vi "Manual.vi"(6 "Cluster":T9={"VISA resource name"="", "baud rate "=9600}, 7 "vi reference":refnum<vi>, 8 "error in (no error)":errorcluster, 9 "IOList_280":T1, 10 "TabCtl Refnum":refnum<vi>, 11 "Manual":T4(tab)) -> (0 "error out":errorcluster, 3 "Out reference":refnum<vi>)   [LabVIEW 2015]
uses:
  Control Button/Exit.ctl
  Control Button/Scanner config.ctl
  Galobal variable_TI.vi
  <vilib>/Instr/_visa.llb/VISA Configure Serial Port (Instr).vi
panel:
  out "Array":string[](array[string])
  out "Byte Lenth":i32
  out "error out 2":errorcluster
  out "Manual DO":bool[](array[boolean])
  in  "Stop":T2
  out "NewVal":T3
  in  "Digital Output":T5
  out "Digital Input":T6
  in  "Home Calling M1":bool
  in  "Stop M1":bool
  in  "Direction M1":bool
  in  "SERVO ON CMD M1":bool
  in  "Speed (mm/s) M1":dbl=10.0
  in  "Travel (mm)M1":dbl=5.0
  out "STM1 Done Bit":bool
  in  "Mode M1":i32(ring)=10178 items=["Finite Samples"=10178, "Continuous Samples"=10123, "Hardware Timed Single Point"=12522]
  out "Waveform Chart":dbl(graph)
  out "Analog Input":T7
  out "Error Status":bool
  in  "Scanner config":T8
  out "Read data":string
  out "Boolean":bool
  # "Fixture Slide servo"
  # "Instruction for Servo motor Operate\n(1)  Switch  ON -OFF  of Fixture Slide servo Brake ON Cmd (P0.19)  \n      from Digital Output tab.\n(2) Switch  ON -OFF  of Fixture Slide Servo Direction Command (P0.20)\n      from Digital Output tab."
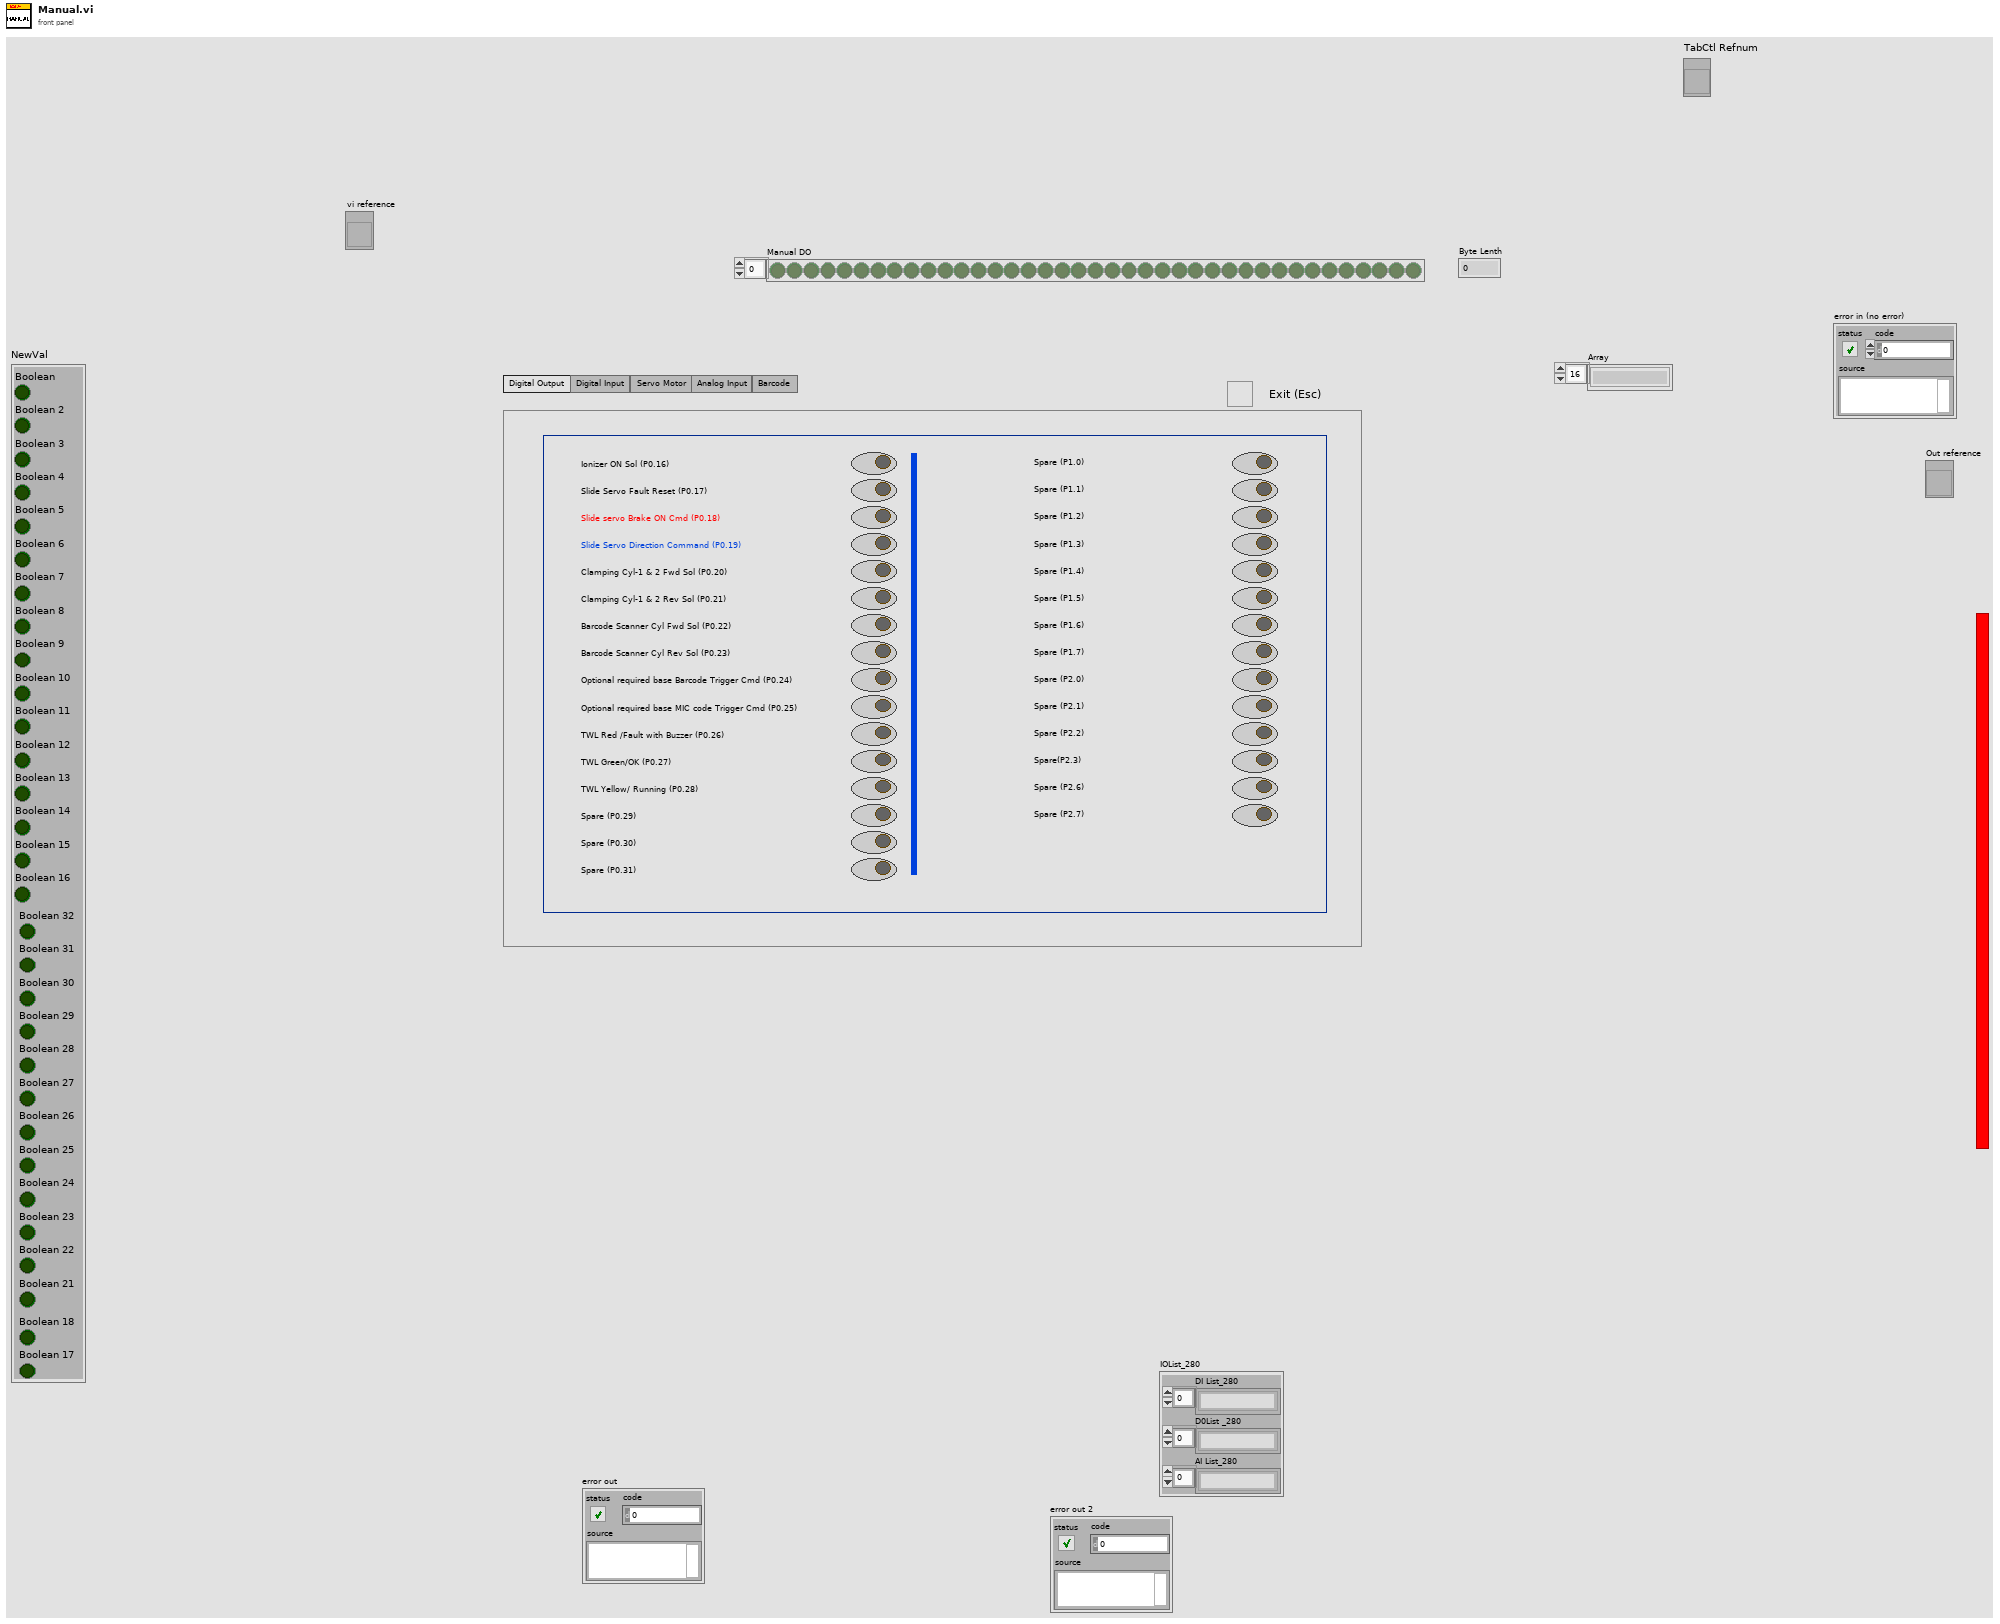
[diagram p1: front panel]
types:
  T1 = cluster{"DI List_280":string[], "D0List _280":string[], "AI List_280":string[]}
  T2 = typedef "Exit.ctl" = bool
  T3 = cluster{"Boolean":bool, "Boolean 2":bool, "Boolean 3":bool, "Boolean 4":bool, "Boolean 5":bool, "Boolean 6":bool, "Boolean 7":bool, "Boolean 8":bool, "Boolean 9":bool, "Boolean 10":bool, "Boolean 11":bool, "Boolean 12":bool, "Boolean 13":bool, "Boolean 14":bool, "Boolean 15":bool, "Boolean 16":bool, "Boolean 17":bool, "Boolean 18":bool, "Boolean 21":bool, "Boolean 22":bool, "Boolean 23":bool, "Boolean 24":bool, "Boolean 25":bool, "Boolean 26":bool, "Boolean 27":bool, "Boolean 28":bool, "Boolean 29":bool, "Boolean 30":bool, "Boolean 31":bool, "Boolean 32":bool}
  T4 = enum32{"Digital Output", "Digital Input", "Servo Motor ", "Analog Input", "Barcode "}
  T5 = cluster{"DO.00":bool, "DO.01":bool, "DO.02":bool, "DO.03":bool, "DO.04":bool, "DO.05":bool, "DO.06":bool, "DO.06":bool, "DO.07":bool, "DO.08":bool, "DO.09":bool, "DO.10":bool, "DO.11":bool, "DO.12":bool, "DO.13":bool, "DO.14":bool, "DO.07 2":bool, "DO.08 2":bool, "DO.09 2":bool, "DO.10 2":bool, "DO.11 2":bool, "DO.12 2":bool, "DO.13 2":bool, "DO.14 2":bool, "DO.00 2":bool, "DO.01 2":bool, "DO.02 2":bool, "DO.03 2":bool, "DO.06 2":bool, "DO.06 3":bool}
  T6 = cluster{"Digital Input":bool, "Digital Input 2":bool, "Digital Input 3":bool, "Digital Input 4":bool, "Digital Input 5":bool, "Digital Input 6":bool, "Digital Input 7":bool, "Digital Input 8":bool, "Digital Input 9":bool, "Digital Input 10":bool, "Digital Input 11":bool, "Digital Input 12":bool, "Digital Input 13":bool, "Digital Input 14":bool, "Digital Input 15":bool, "Digital Input 16":bool, "Digital Input 17":bool, "Digital Input 18":bool, "Digital Input 19":bool, "Digital Input 20":bool, "Digital Input 21":bool, "Digital Input 22":bool, "Digital Input 23":bool, "Digital Input 24":bool, "Digital Input 25":bool, "Digital Input 26":bool, "Digital Input 27":bool, "Digital Input 28":bool, "Digital Input 29":bool, "Digital Input 30":bool, "Digital Input 31":bool, "Digital Input 32":bool, "Digital Input 33":bool, "Digital Input 34":bool, "Digital Input 35":bool, "Digital Input 36":bool, "Digital Input 37":bool, "Digital Input 38":bool, "Digital Input 39":bool}
  T7 = cluster{"Analog Data":dbl, "Analog Data 2":dbl, "Analog Data 3":dbl, "Analog Data 4":dbl, "Analog Data 5":dbl, "Analog Data 6":dbl}
  T8 = typedef "Scanner config.ctl" = bool
  T9 = cluster{"VISA resource name":refnum<visa-resource-name>, "baud rate ":u32}
  T10 = cluster{"Analoge Input[0]":dbl, "Analoge Input[1]":dbl, "Analoge Input[2]":dbl, "Analoge Input[3]":dbl, "Analoge Input[4]":dbl, "Analoge Input[5]":dbl}
  T11 = cluster{"Digital input[0]":bool, "Digital input[1]":bool, "Digital input[2]":bool, "Digital input[3]":bool, "Digital input[4]":bool, "Digital input[5]":bool, "Digital input[6]":bool, "Digital input[7]":bool, "Digital input[8]":bool, "Digital input[9]":bool, "Digital input[10]":bool, "Digital input[11]":bool, "Digital input[12]":bool, "Digital input[13]":bool, "Digital input[14]":bool, "Digital input[15]":bool, "Digital input[16]":bool, "Digital input[17]":bool, "Digital input[18]":bool, "Digital input[19]":bool, "Digital input[20]":bool, "Digital input[21]":bool, "Digital input[22]":bool, "Digital input[23]":bool, "Digital input[24]":bool, "Digital input[25]":bool, "Digital input[26]":bool, "Digital input[27]":bool, "Digital input[28]":bool, "Digital input[29]":bool, "Digital input[30]":bool, "Digital input[31]":bool, "Digital input[32]":bool, "Digital input[33]":bool, "Digital input[34]":bool, "Digital input[35]":bool, "Digital input[36]":bool, "Digital input[37]":bool, "Digital input[38]":bool}
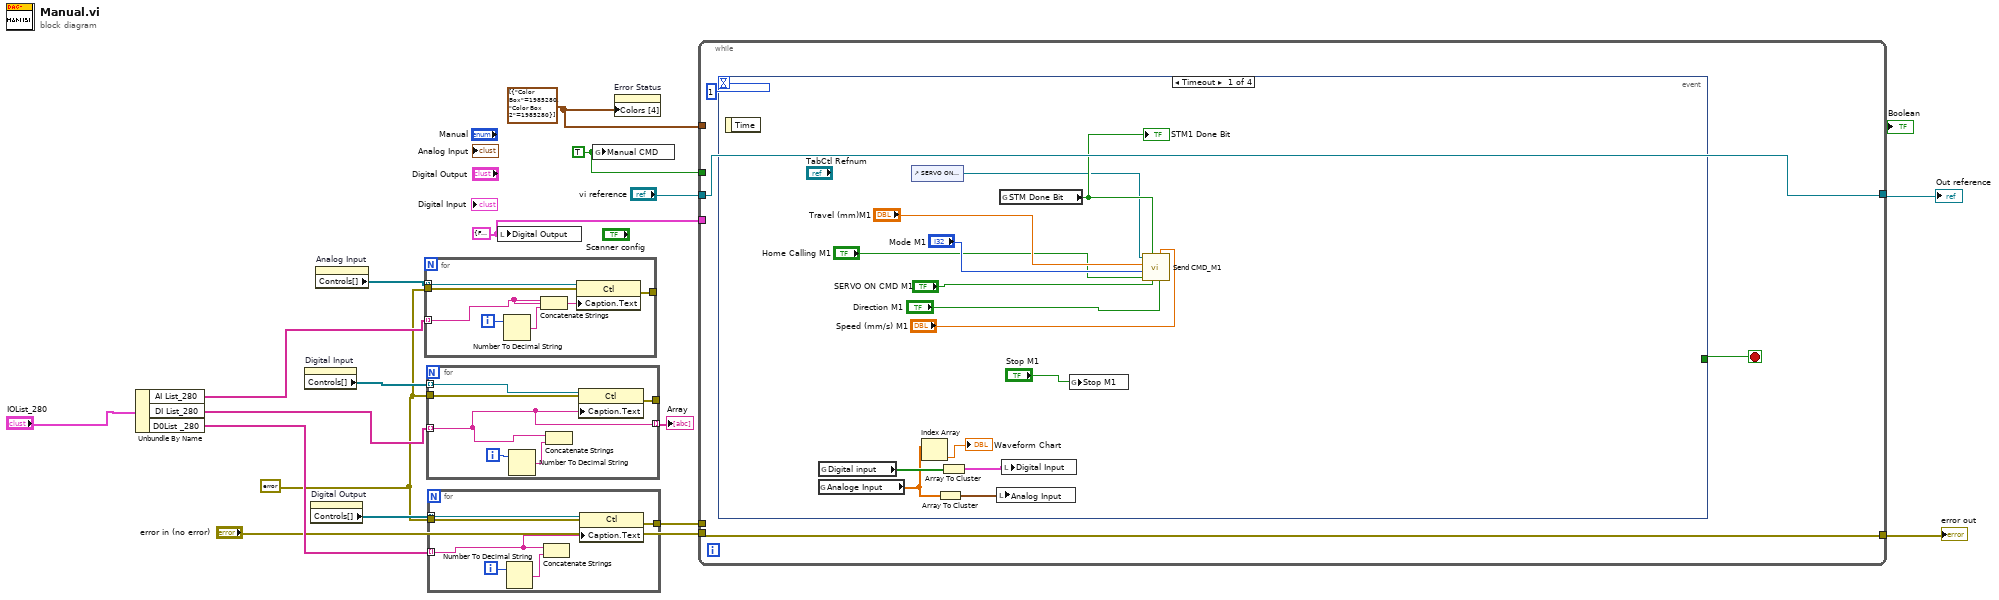
[diagram p0: block diagram]
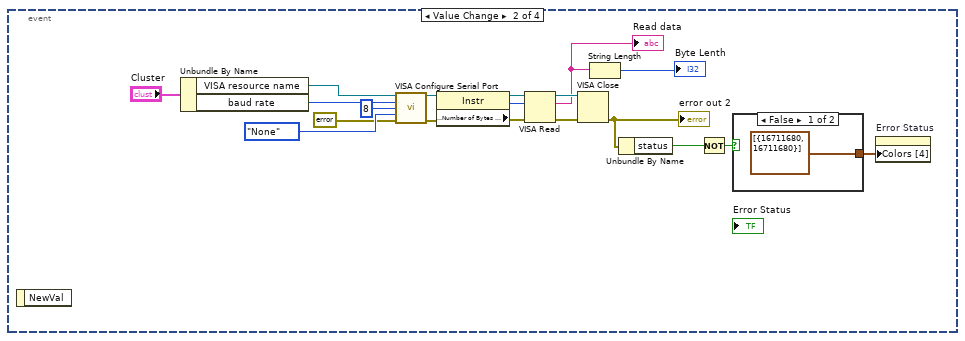
[diagram p2: hidden frame]
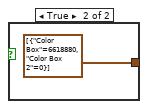
[diagram p3: hidden frame]
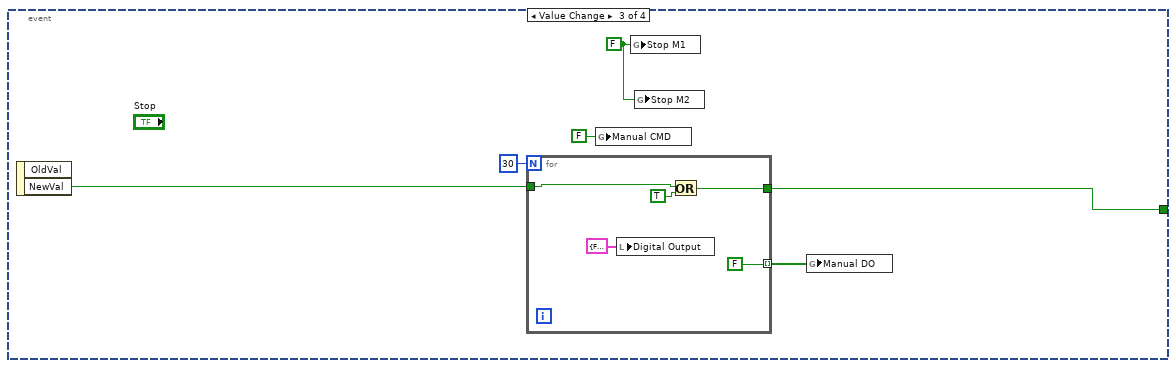
[diagram p4: hidden frame]
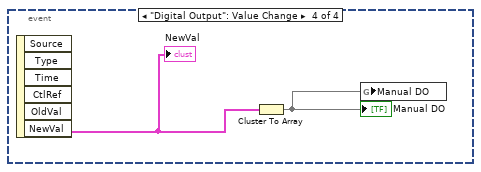
[diagram p5: hidden frame]
diagram:
  w1 = T5 {"DO.00"=FALSE, "DO.01"=FALSE, "DO.02"=FALSE, "DO.03"=FALSE, "DO.04"=FALSE, "DO.05"=FALSE, "DO.06"=FALSE, "DO.06"=FALSE, "DO.07"=FALSE, "DO.08"=FALSE, "DO.09"=FALSE, "DO.10"=FALSE, "DO.11"=FALSE, "DO.12"=FALSE, "DO.13"=FALSE, "DO.14"=FALSE, "DO.07 2"=FALSE, "DO.08 2"=FALSE, "DO.09 2"=FALSE, "DO.10 2"=FALSE, "DO.11 2"=FALSE, "DO.12 2"=FALSE, "DO.13 2"=FALSE, "DO.14 2"=FALSE, "DO.00 2"=FALSE, "DO.01 2"=FALSE, "DO.02 2"=FALSE, "DO.03 2"=FALSE, "DO.06 2"=FALSE, "DO.06 3"=FALSE} ("Digital Output")
  w4 = errorcluster {"status"=FALSE, "code"=0, "source"=""} ("error in (no error)")
  w7 = cluster{"Color Box":u32, "Color Box 2":u32}[] [{"Color Box"=1985280, "Color Box 2"=1985280}] ("Colors [4]")
  w13 = TRUE ("Manual CMD")
  n1 = Unbundle By Name("IOList_280") -> ("AI List_280"=w8:string[], "DI List_280"=w10:string[], "D0List _280"=w12:string[])
  n2 = property on="Digital Input" class="Clust (strict)"() -> ("Controls[]"=w11:refnum<vi>[])  [unwired: 2 in, 2 out]
  n3 = property on="Digital Output" class="Clust (strict)"() -> ("Controls[]"=w16:refnum<vi>[])  [unwired: 2 in, 2 out]
  n4 = property on="Analog Input" class="Clust (strict)"() -> ("Controls[]"=w9:refnum<vi>[])  [unwired: 2 in, 2 out]
  n5 = for {
    tunnel: w9 -> [w23] mode=indexing
    tunnel: [w21] -> _
    tunnel: w4 -> [w19]
    tunnel: w8 -> [w18] mode=indexing
    i -> [w22]
    n6 = Number To Decimal String(number=w22) -> (decimal integer string=w20:string)  [unwired: 1 in]
    n7 = Concatenate Strings(w18, w20) -> ()  [unwired: 1 out]
    n8 = property class="Ctl"(reference=w23, error in=w19, "Caption.Text"=w18) -> (error out=w21:errorcluster)  [unwired: 1 out]
  }
  n9 = for {
    tunnel: w11 -> [w29] mode=indexing
    tunnel: [w27] -> _
    tunnel: w4 -> [w25]
    tunnel: w10 -> [w24] mode=indexing
    tunnel: [w24] -> w5 mode=indexing
    i -> [w28]
    n10 = Number To Decimal String(number=w28) -> (decimal integer string=w26:string)  [unwired: 1 in]
    n11 = Concatenate Strings(w24, w26) -> ()  [unwired: 1 out]
    n12 = property class="Ctl"(reference=w29, error in=w25, "Caption.Text"=w24) -> (error out=w27:errorcluster)  [unwired: 1 out]
  }
  "Array" <- w5
  n13 = for {
    tunnel: w16 -> [w35] mode=indexing
    tunnel: [w33] -> w17
    tunnel: w4 -> [w31]
    tunnel: w12 -> [w30] mode=indexing
    i -> [w34]
    n14 = Number To Decimal String(number=w34) -> (decimal integer string=w32:string)  [unwired: 1 in]
    n15 = Concatenate Strings(w30, w32) -> ()  [unwired: 1 out]
    n16 = property class="Ctl"(reference=w35, error in=w31, "Caption.Text"=w30) -> (error out=w33:errorcluster)  [unwired: 1 out]
  }
  n17 = local write "Digital Output"(w1) -> ()
  n18 = global write "Galobal variable_TI.vi" "Manual CMD"(w13) -> ()
  n19 = property on="Error Status" class="Bool (strict)"("Colors [4]"=w7) -> ()  [unwired: 2 in, 2 out]
  n20 = while {
    tunnel: w17 -> [_]
    tunnel: [w37] -> w15
    tunnel: "vi reference" -> [w38]
    tunnel: [w38] -> w14
    tunnel: w13 -> [_]
    tunnel: w7 -> [_]
    tunnel: "error in (no error)" -> [w37]
    tunnel: w1 -> [_]
    stop <- w36 stop-if-true
    n21 = event shown="[0] Timeout" {
      selector: _ -> [_ _ _ _]
      dyn-events: _ -> [_ _ _ _]
      timeout: 1 -> [_ _ _ _]
      tunnel: [_ _ w75 _] -> w36
      event Timeout {
        n22 = event-data() -> ()  [unwired: 1 in, 1 out]
        n23 = global read "Galobal variable_TI.vi" "Analoge Input"() -> (w48:dbl[])
        n24 = global read "Galobal variable_TI.vi" "Digital input"() -> (w52:bool[])
        n25 = control-ref of="SERVO ON CMD M1"() -> (w40:refnum<vi>)
        n26 = Index Array(array=w48) -> (element=→"Waveform Chart":dbl)  [unwired: 1 in]
        n27 = Array To Cluster(array=w48) -> (cluster=w50:T10)
        n28 = Array To Cluster(array=w52) -> (cluster=w51:T11)
        n29 = local write "Analog Input"(w50) -> ()
        n30 = global read "Galobal variable_TI.vi" "STM Done Bit"() -> (w49:bool)
        "STM1 Done Bit" <- w49
        n31 = local write "Digital Input"(w51) -> ()
        n32 = global write "Galobal variable_TI.vi" "Stop M1"("Stop M1") -> ()
        n33 = call "Send CMD_M1.vi"("Direction M1"="Direction M1", "Speed (mm/s) M1"="Speed (mm/s) M1", "SERVO ON CMD M1"="SERVO ON CMD M1", "STM Done Bit"=w49, "Home Calling M1"="Home Calling M1", "Mode M1"="Mode M1", "Travel (mm)M1"="Travel (mm)M1", "Bool Refnum"=w40) -> ()  [unwired: 4 in]
      }
      event Value Change {
        n34 = event-data() -> ()  [unwired: 1 in, 1 out]
        n35 = Unbundle By Name("Cluster") -> ("VISA resource name"=w72:refnum<visa-resource-name>, "baud rate"=w71:u32)
        n36 = call-poly "VISA Configure Serial Port"("VISA resource name"=w72, "baud rate (9600)"=w71, "data bits (8)"=u16 8, "parity (0:none)"=enum16{"None", "Odd", "Even", "Mark", "Space"}."None", "error in (no error)"=errorcluster {"status"=FALSE, "code"=0, "source"=""} ("error in (no error) 2")) -> ("VISA resource name out"=w70:refnum<visa-resource-name>, "error out"=w68:errorcluster)  [unwired: 9 in]
        n37 = property class="Instr"(reference=w70, error in=w68) -> (reference out=w69:refnum<visa-resource-name>, error out=w67:errorcluster, "Serial Settings:Number of Bytes at Serial Port"=w66:u32)
        n38 = VISA Read(VISA resource name=w69, byte count=w66, error in (no error)=w67) -> (VISA resource name out=w64:refnum<visa-resource-name>, read buffer=w62:string, error out=w63:errorcluster)  [unwired: 1 out]
        "Read data" <- w62
        n39 = VISA Close(VISA resource name=w64, error in (no error)=w63) -> (error out=w60:errorcluster)
        "error out 2" <- w60
        n40 = String Length(string=w62) -> (length=→"Byte Lenth":i32)
        n41 = Unbundle By Name(w60) -> ("status"=w59:bool)
        n42 = Not(x=w59) -> (.not. x?=w57:bool)
        n43 = case shown="False" w57 {
          tunnel: [cluster{"Color Box":u32, "Color Box 2":u32}[] [{"Color Box"=16711680, "Color Box 2"=16711680}] ("Colors [4]") cluster{"Color Box":u32, "Color Box 2":u32}[] [{"Color Box"=6618880, "Color Box 2"=0}] ("Colors [4]")] -> w58
          frame False {
          }
          frame True {
          }
        }
        n44 = property on="Error Status" class="Bool (strict)"("Colors [4]"=w58) -> ()  [unwired: 2 in, 2 out]
      }
      event Value Change {
        w79 = FALSE ("Stop M1")
        n45 = event-data() -> ("NewVal"=w76:T2)  [unwired: 1 in, 1 out]
        n46 = for {
          N: 30 -> [_]
          tunnel: [FALSE] -> w78 mode=indexing
          tunnel: w76 -> [w83]
          tunnel: [w82] -> w75
          n47 = local write "Digital Output"(T5 {"DO.00"=FALSE, "DO.01"=FALSE, "DO.02"=FALSE, "DO.03"=FALSE, "DO.04"=FALSE, "DO.05"=FALSE, "DO.06"=FALSE, "DO.06"=FALSE, "DO.07"=FALSE, "DO.08"=FALSE, "DO.09"=FALSE, "DO.10"=FALSE, "DO.11"=FALSE, "DO.12"=FALSE, "DO.13"=FALSE, "DO.14"=FALSE, "DO.07 2"=FALSE, "DO.08 2"=FALSE, "DO.09 2"=FALSE, "DO.10 2"=FALSE, "DO.11 2"=FALSE, "DO.12 2"=FALSE, "DO.13 2"=FALSE, "DO.14 2"=FALSE, "DO.00 2"=FALSE, "DO.01 2"=FALSE, "DO.02 2"=FALSE, "DO.03 2"=FALSE, "DO.06 2"=FALSE, "DO.06 3"=FALSE} ("Digital Output")) -> ()
          n48 = Or(x=w83, y=TRUE) -> (x .or. y?=w82:T2)
        }
        n49 = global write "Galobal variable_TI.vi" "Manual CMD"(FALSE ("Manual CMD")) -> ()
        n50 = global write "Galobal variable_TI.vi" "Stop M1"(w79) -> ()
        n51 = global write "Galobal variable_TI.vi" "Stop M2"(w79) -> ()
        n52 = global write "Galobal variable_TI.vi" "Manual DO"(w78) -> ()
      }
      event "Digital Output": Value Change {
        n53 = event-data() -> ("NewVal"=w86:T5)  [unwired: 1 in, 5 out]
        "NewVal" <- w86
        n54 = Cluster To Array(cluster=w86) -> (array=w87:bool[])
        "Manual DO" <- w87
        n55 = global write "Galobal variable_TI.vi" "Manual DO"(w87) -> ()
      }
    }
  }
  "error out" <- w15
  "Out reference" <- w14
